vi "Import Transactions from File.vi"(8 "error in (no error)":errorcluster) -> (0 "error out":errorcluster, 3 "Importing Transactions":refnum<class "Statement.lvclass">)   [LabVIEW 2018]
uses:
  classes/Statement/Statement.lvclass
  <vilib>/Utility/sysdir.llb/System Directory Type.ctl
  classes/Banking Statement/Banking Statement.lvclass
  C:/Users/jtipps/Documents/Filthy-Lucre-Budgetizer/source/support/classes/Statement/Statement.lvclass
  classes/Credit Statement/Credit Statement.lvclass
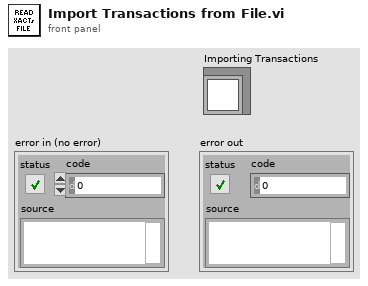
[diagram p1: front panel]
types:
  T1 = typedef "System Directory Type.ctl" = i32
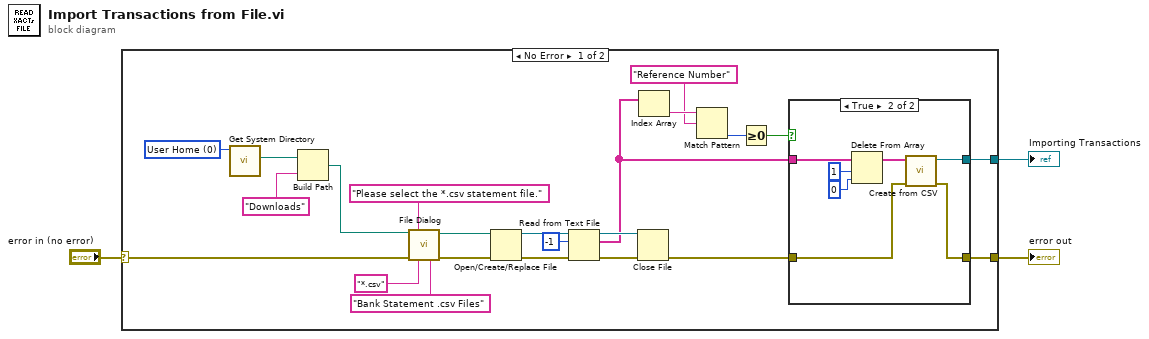
[diagram p0: block diagram]
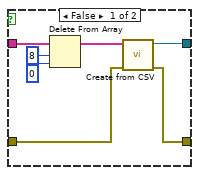
[diagram p2: hidden frame]
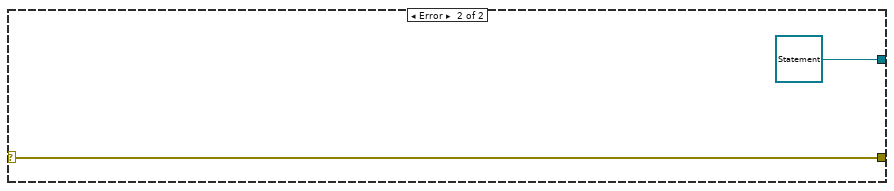
[diagram p3: hidden frame]
diagram:
  n1 = case shown="No Error" "error in (no error)" {
    selector: "error in (no error)" -> [w12 w42]
    tunnel: [w10 w42] -> w3
    tunnel: [w9 refnum<class "Statement.lvclass"> refnum ("Statement")] -> w1
    frame No Error {
      w16 = T1 0 items=["User Home"=0, "User Desktop"=1, "User Documents"=2, "User Application Data"=3, "User Preferences"=4, "User Temporary"=5, "Public Documents"=6, "Public Application Data"=7, "Public Preferences"=8, "Public Cache"=13, "System Core Libraries"=9, "System Installed Libraries"=10, "Application Files"=11, "Boot Volume Root"=12] ("system directory type")
      n2 = call <vilib>:"Get System Directory.vi"("system directory type"=w16) -> ("system directory"=w15:path)  [unwired: 10 in]
      n3 = Build Path(base path=w15, name or relative path="Downloads") -> (appended path=w13:path)
      n4 = call "File Dialog"("start path"=w13, "prompt"="Please select the *.csv statement file.", "error in"=w12, "pattern (all files)"="*.csv", "pattern label"="Bank Statement .csv Files") -> ("selected path"=w18:path, "error out"=w17:errorcluster)  [unwired: 2 in, 7 out]
      n5 = Open/Create/Replace File(file path (use dialog)=w18, error in=w17) -> (refnum out=w23:refnum<file>, error out=w22:errorcluster)  [unwired: 5 out]
      n6 = Read from Text File(file (use dialog)=w23, count=-1, error in=w22) -> (refnum out=w20:refnum<file>, text=w8:string[], error out=w21:errorcluster)  [unwired: 2 out]
      n7 = Close File(refnum=w20, error in=w21) -> (error out=w11:errorcluster)  [unwired: 1 out]
      n8 = Index Array(array=w8) -> (element=w7:string)  [unwired: 1 in]
      n9 = Match Pattern(string=w7, regular expression="Reference Number") -> (offset past match=w5:i32)  [unwired: 1 in, 3 out]
      n10 = Greater Or Equal To 0?(x=w5) -> (x >= 0?=w4:bool)
      n11 = case shown="True" w4 {
        tunnel: w11 -> [w31 w35]
        tunnel: [w30 w34] -> w10
        tunnel: [w28 w36] -> w9
        tunnel: w8 -> [w27 w38]
        frame False {
          n12 = Delete From Array(array=w27, length=8, index=0) -> (array with subset deleted=w29:string[])  [unwired: 1 out]
          n13 = call "Create from CSV.vi"("error in (no error)"=w31, "CSV Entries"=w29) -> ("error out"=w30:errorcluster, "Banking Statement out"=w28:refnum<class "Banking Statement.lvclass">)  [unwired: 8 in]
        }
        frame True {
          n14 = Delete From Array(array=w38, length=1, index=0) -> (array with subset deleted=w37:string[])  [unwired: 1 out]
          n15 = call "Create from CSV.vi"("error in (no error)"=w35, "CSV Entries"=w37) -> ("error out"=w34:errorcluster, "Credit Statement out"=w36:refnum<class "Credit Statement.lvclass">)  [unwired: 8 in]
        }
      }
    }
    frame Error {
    }
  }
  "error out" <- w3
  "Importing Transactions" <- w1
